vi "My Nonlinear Curve Fit Intervals.vi"(0 "Y":dbl[](array[numeric]), 1 "confidence level":dbl=0.95, 2 "f(x,a)":T1, 3 "data":variant, 5 "X":dbl[](array[numeric]), 7 "Weight":dbl[](array[numeric]), 9 "best fit parameters":dbl[](array[numeric]), 11 "error in (no error)":errorcluster) -> (10 "delta best fit parameters":dbl[](array[numeric]), 15 "error out":errorcluster)   [LabVIEW 2021, in "Fits.lvlib"]
uses:
  Fits.lvlib
  <vilib>/gmath/NumericalOptimization/LM model function reference.ctl
  <vilib>/gmath/NumericalOptimization/LM_output select.ctl
  <vilib>/Analysis/baseanly.llb/Real A x B.vi
  <vilib>/Analysis/NI_AALPro.lvlib
  <vilib>/gmath/NI_Gmath.lvlib
  <vilib>/Analysis/NI_AALBase.lvlib
  Error/Error.lvlib
panel:
  # "see the AlliGator License on the block diagram (Ctrl+E or Window:Show Block Diagram)"
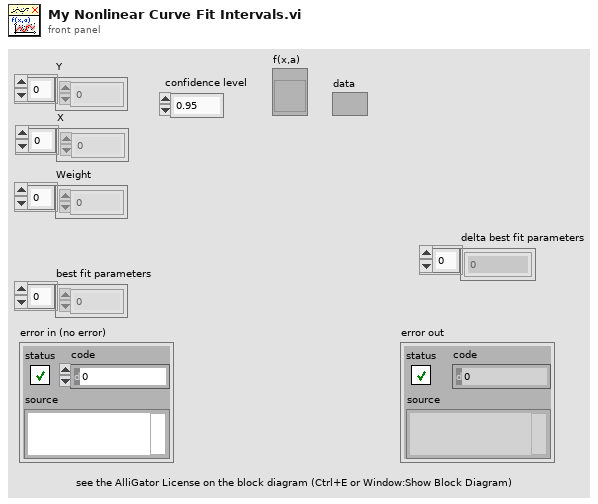
[diagram p1: front panel]
types:
  T1 = typedef "NI_Gmath.lvlib/LM model function reference.ctl" = refnum<vi>
  T2 = typedef "NI_Gmath.lvlib/LM_output select.ctl" = cluster{"model function":bool, "gradient":bool}
  T3 = typedef "NI_Matrix.lvlib/RealMatrix.ctl" = dbl[][]
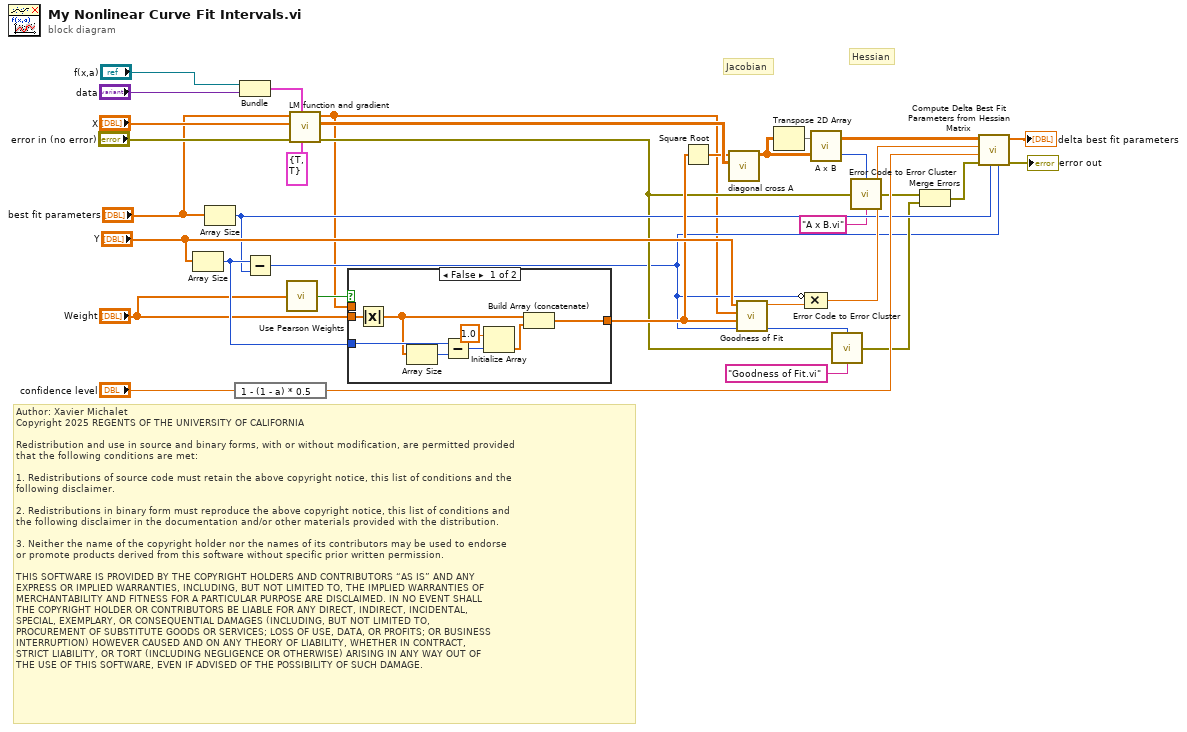
[diagram p0: block diagram]
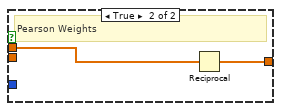
[diagram p2: hidden frame]
diagram:
  # "Author: Xavier Michalet\nCopyright 2025 REGENTS OF THE UNIVERSITY OF CALIFORNIA\n\nRedistribution and use in source and binary forms, with or without modification, are permitted provided\nthat the following conditions are met:\n\n1. Redistributions of source code must retain the above copyright notice, this list of conditions and the\nfollowing disclaimer.\n\n2. Redistributions in binary form must reproduce the above copyright notice, this list of conditions and\nthe following disclaimer in the documentation and/or other materials provided with the distribution.\n\n3. Neither the name of the copyright holder nor the names of its contributors may be used to endorse \nor promote products derived from this software without specific prior written permission.\n\nTHIS SOFTWARE IS PROVIDED BY THE COPYRIGHT HOLDERS AND CONTRIBUTORS “AS IS” AND ANY \nEXPRESS OR IMPLIED WARRANTIES, INCLUDING, BUT NOT LIMITED TO, THE IMPLIED WARRANTIES OF\nMERCHANTABILITY AND FITNESS FOR A PARTICULAR PURPOSE ARE DISCLAIMED. IN NO EVENT SHALL\nTHE COPYRIGHT HOLDER OR CONTRIBUTORS BE LIABLE FOR ANY DIRECT, INDIRECT, INCIDENTAL, \nSPECIAL, EXEMPLARY, OR CONSEQUENTIAL DAMAGES (INCLUDING, BUT NOT LIMITED TO, \nPROCUREMENT OF SUBSTITUTE GOODS OR SERVICES; LOSS OF USE, DATA, OR PROFITS; OR BUSINESS\nINTERRUPTION) HOWEVER CAUSED AND ON ANY THEORY OF LIABILITY, WHETHER IN CONTRACT, \nSTRICT LIABILITY, OR TORT (INCLUDING NEGLIGENCE OR OTHERWISE) ARISING IN ANY WAY OUT OF\nTHE USE OF THIS SOFTWARE, EVEN IF ADVISED OF THE POSSIBILITY OF SUCH DAMAGE."
  # "Hessian"
  # "Jacobian"
  n1 = Array Size(array="Y") -> (size(s)=w21:i32)
  n2 = Array Size(array="best fit parameters") -> (size(s)=w14:i32)
  n3 = expression code="1 - (1 - a) * 0.5"("confidence level") -> (w16:dbl)
  n4 = Bundle("f(x,a)"="f(x,a)", "data"="data") -> (w30:cluster{"f(x,a)":T1, "data":variant})  [unwired: 1 in]
  n5 = Subtract(x=w21, y=w14) -> (x-y=w6:i32)
  n6 = call "Use Pearson Weights.vi"("Weight"="Weight") -> ("Use Pearson Weight"=w2:bool)
  n7 = call <vilib>:"LM function and gradient.vi"("output control"=T2 {"model function"=TRUE, "gradient"=TRUE}, "model function"=w30, "error in (no error)"="error in (no error)", "X"="X", "a"="best fit parameters") -> ("error out"=w11:errorcluster, "gradient"=w20:dbl[][], "f(X)"=w1:dbl[])  [unwired: 3 in, 1 out]
  n8 = case shown="False" w2 {
    tunnel: "Weight" -> [w38 _]
    tunnel: [w37 w43] -> w22
    tunnel: w21 -> [w36 _]
    tunnel: w1 -> [_ w44]
    frame False {
      n9 = Absolute Value(x=w38) -> (abs(x)=w35:dbl[])
      n10 = Array Size(array=w35) -> (size(s)=w41:i32)
      n11 = Subtract(x=w36, y=w41) -> (x-y=w39:i32)
      n12 = Initialize Array(1.0, w39) -> (w40:dbl[])
      n13 = Build Array (concatenate)(w35, w40) -> (w37:dbl[])
    }
    frame True {
      # "Pearson Weights"
      n14 = Reciprocal(x=w44) -> (1/x=w43:dbl[])
    }
  }
  n15 = Square Root(x=w22) -> (sqrt(x)=w19:dbl[])
  n16 = call <vilib>:"diagonal cross A.vi"("A"=w20, "diagonal"=w19) -> ("diagonalxA"=w18:T3)  [unwired: 9 in]
  n17 = call <vilib>:"Goodness of Fit.vi"("degree of freedom"=w6, "Weight"=w22, "Best Fit"=w1, "Y"="Y") -> ("error"=w12:i32, "SSE"=w17:dbl)  [unwired: 4 in, 2 out]
  n18 = Transpose 2D Array(2D array=w18) -> (transposed array=w26:T3)
  n19 = Compound Arithmetic op=MULTIPLY(invert w6, w17) -> (w15:dbl)
  n20 = call-poly <vilib>:"A x B.vi"("B"=w18, "A"=w26) -> ("error"=w13:i32, "A x B"=w25:T3)
  n21 = call "Error Code to Error Cluster.vi"("Error Code"=w12, "Error Source"="Goodness of Fit.vi", "Error In"=w11) -> ("Error Out"=w8:errorcluster)  [unwired: 12 in]
  n22 = call "Error Code to Error Cluster.vi"("Error Code"=w13, "Error Source"="A x B.vi", "Error In"=w11) -> ("Error Out"=w10:errorcluster)  [unwired: 12 in]
  n23 = Merge Errors(w10, w8) -> (w9:errorcluster)
  n24 = call "Compute Delta Best Fit Parameters from Hessian Matrix.vi"("# Degrees of Freedom"=w6, "# Parameters"=w14, "Error In"=w9, "CL Parameter"=w16, "Chi2"=w15, "Hessian"=w25) -> ("Error Out"=→"error out":errorcluster, "Delta Best Fit Parameters"=→"delta best fit parameters":dbl[])  [unwired: 4 in]
